vi "Save CRT data to file.vi"(5 "GPS data granularity (minutes)":refnum<vi>, 6 "Hitrate save info":T2, 7 "ROB data granularity (minutes)":refnum<vi>, 8 "error in":errorcluster, 9 "Run ID":refnum<vi>, 10 "ROB Info cluster":refnum<vi>, 11 "HDF5 data file":refnum<vi>) -> (0 "error out":errorcluster)   [LabVIEW 2016]
uses:
  Typedefs/Hit chart cluster refnum.ctl
  Typedefs/CoincidencesToSave.ctl
  Typedefs/CoincidenceWithGPSformat.ctl
  Global Variables/take CRT data.vi
  <vilib>/addons/h5labview2/group/H5G.lvlib
  <vilib>/addons/h5labview2/dataset/H5D.lvlib
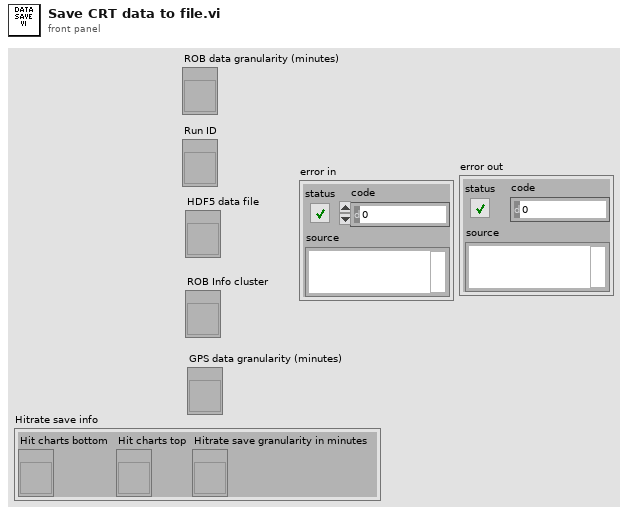
[diagram p1: front panel]
types:
  T1 = typedef "Hit chart cluster refnum.ctl" = refnum<vi>
  T2 = cluster{"Hit charts bottom":T1, "Hit charts top":T1, "Hitrate save granularity in minutes":refnum<vi>}
  T3 = typedef "CoincidenceWithGPSformat.ctl" = cluster{"Low-res hit time":u32, "Hi-res hit time":u32, "Secondary ID":i8, "DeltaT":i32, "Primary ID":i8}
  T4 = typedef "CoincidencesToSave.ctl" = T3[]
  T5 = cluster{"Timestamp":u32, "Fix quality":i8, "Satelites":i8}
  T6 = enum16{"insertPPS", "insertUTC", "read", "initiate"}
  T7 = typedef "hid_t.ctl" = i32
  T8 = cluster{"Pixel":i8, "Hi res hit time":u32, "Low res hit time":u32, "DeltaT":i16}[]
  T9 = typedef "HitChart.ctl" = cluster{"Waveform Chart":cluster{"Coincidences":dbl, "Non-coincidences":dbl, "Ratio":dbl, "Total hits":dbl}[], "Last update timestamp":timestamp, "Resolution(s)":dbl, "nondisplayed coincs":i32, "nondisplayed noncoincs":i32, "Last upd":i64, "ID":i8}
  T10 = cluster{"Waveform Chart":T9, "Waveform Chart 2":T9, "Waveform Chart 3":T9, "Waveform Chart 4":T9, "Waveform Chart 5":T9, "Waveform Chart 6":T9, "Waveform Chart 7":T9, "Waveform Chart 8":T9}
  T11 = cluster{"timestamp":u32, "ch0":dbl, "ch1":dbl, "ch2":dbl, "ch3":dbl, "ch4":dbl, "ch5":dbl, "ch6":dbl, "ch7":dbl, "ch8":dbl, "ch9":dbl, "ch10":dbl, "ch11":dbl, "ch12":dbl, "ch13":dbl, "ch14":dbl, "ch15":dbl}[]
  T12 = cluster{"Timestamp":u32, "Fix quality":i8, "Satelites":i8}[]
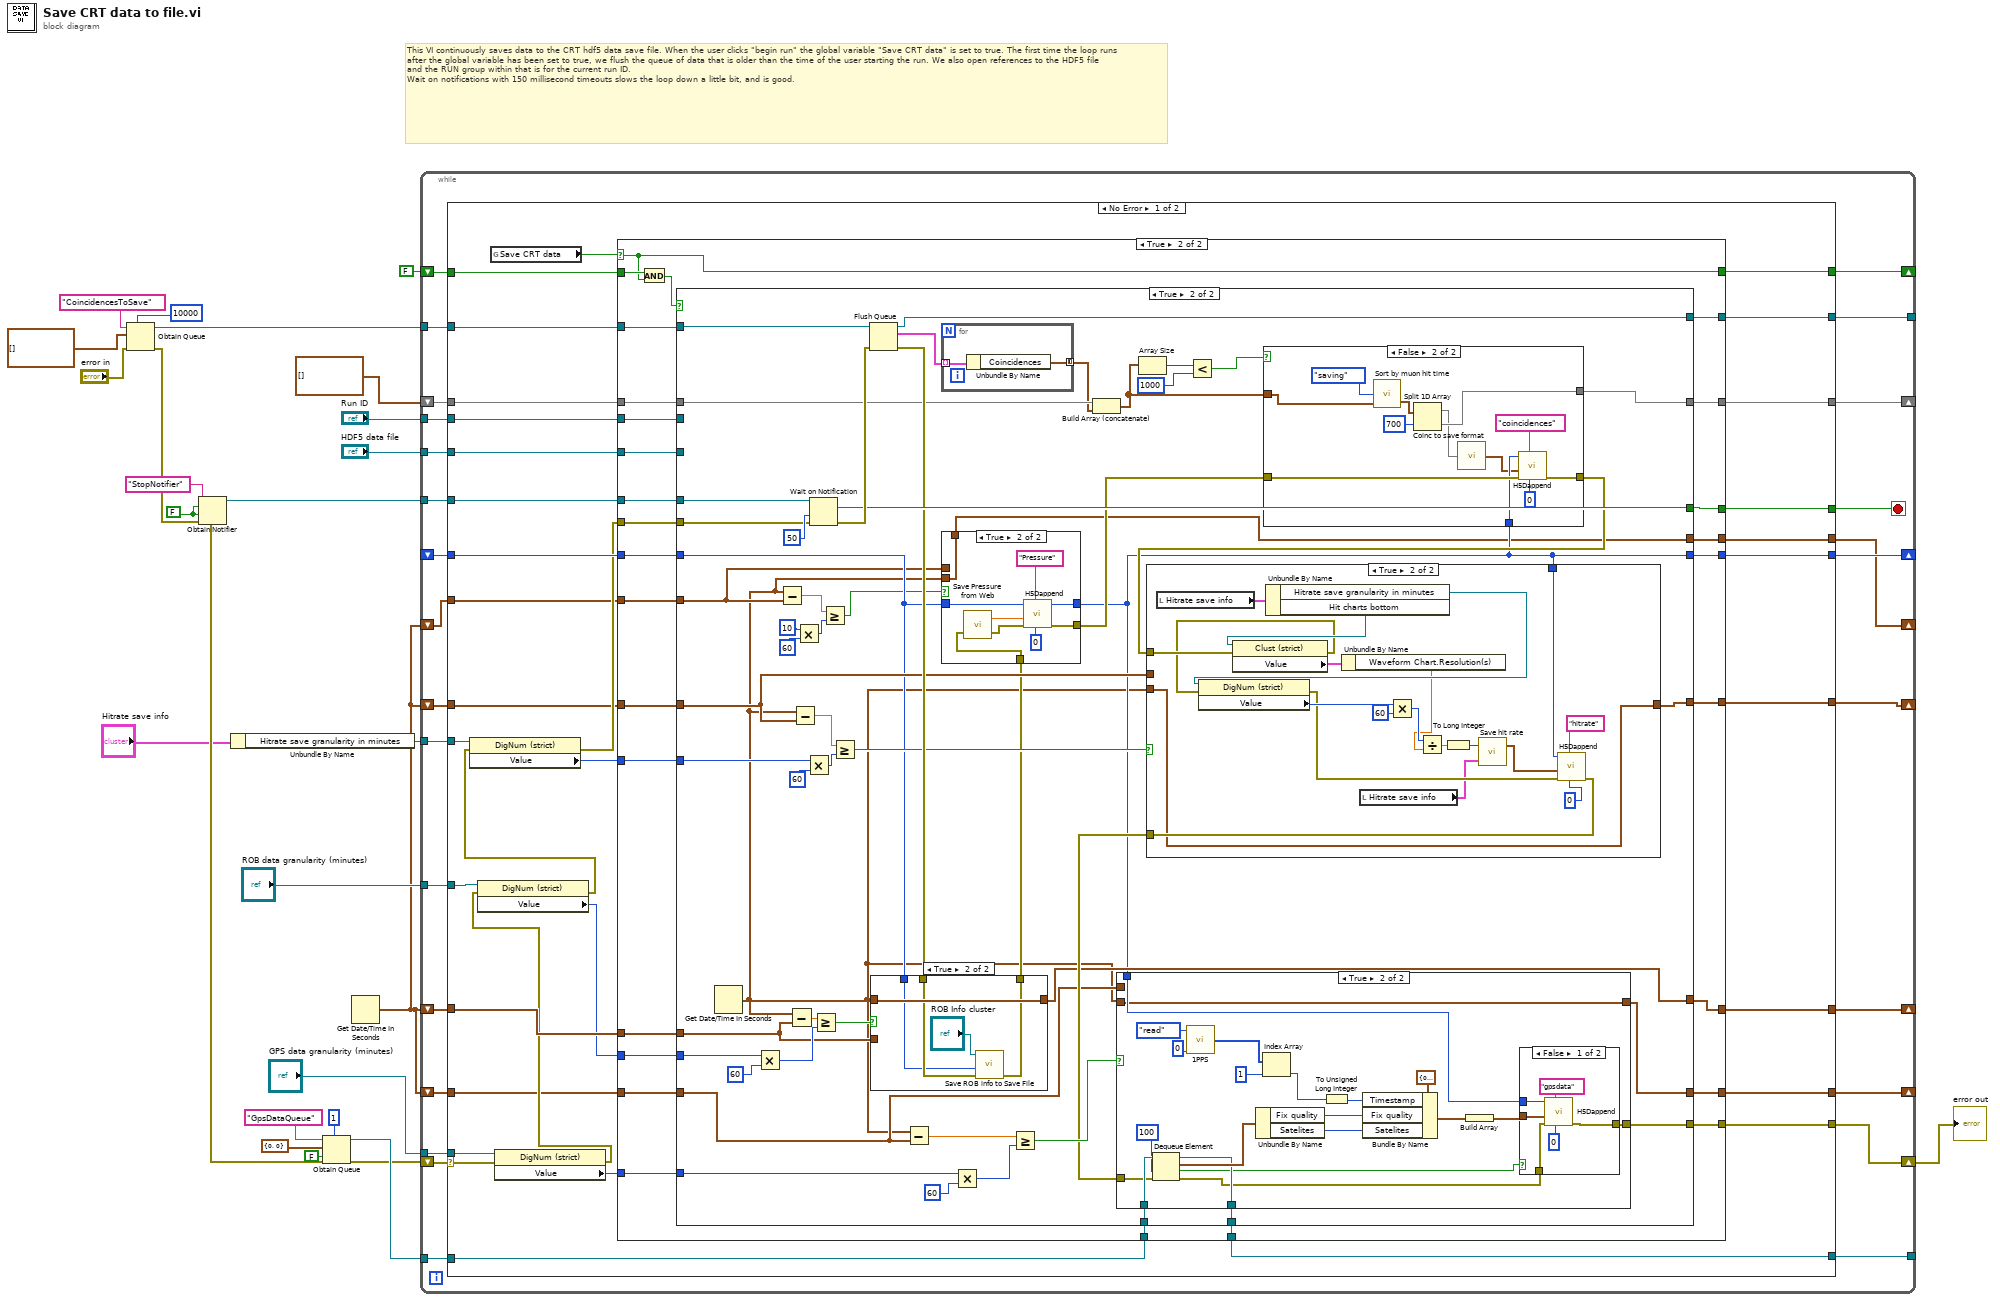
[diagram p0: block diagram]
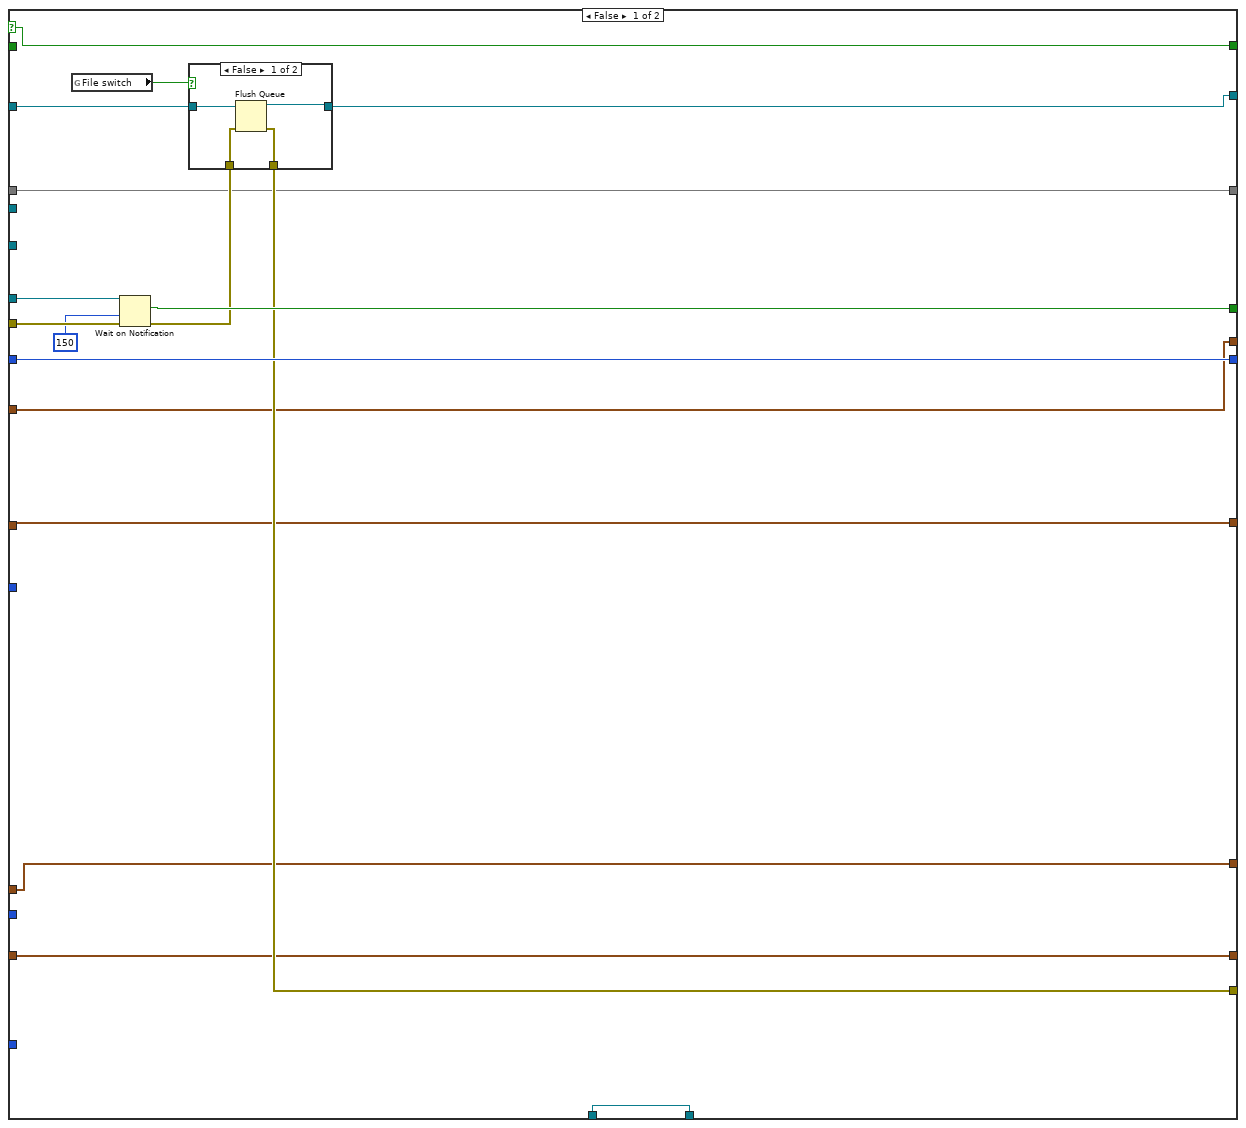
[diagram p2: hidden frame]
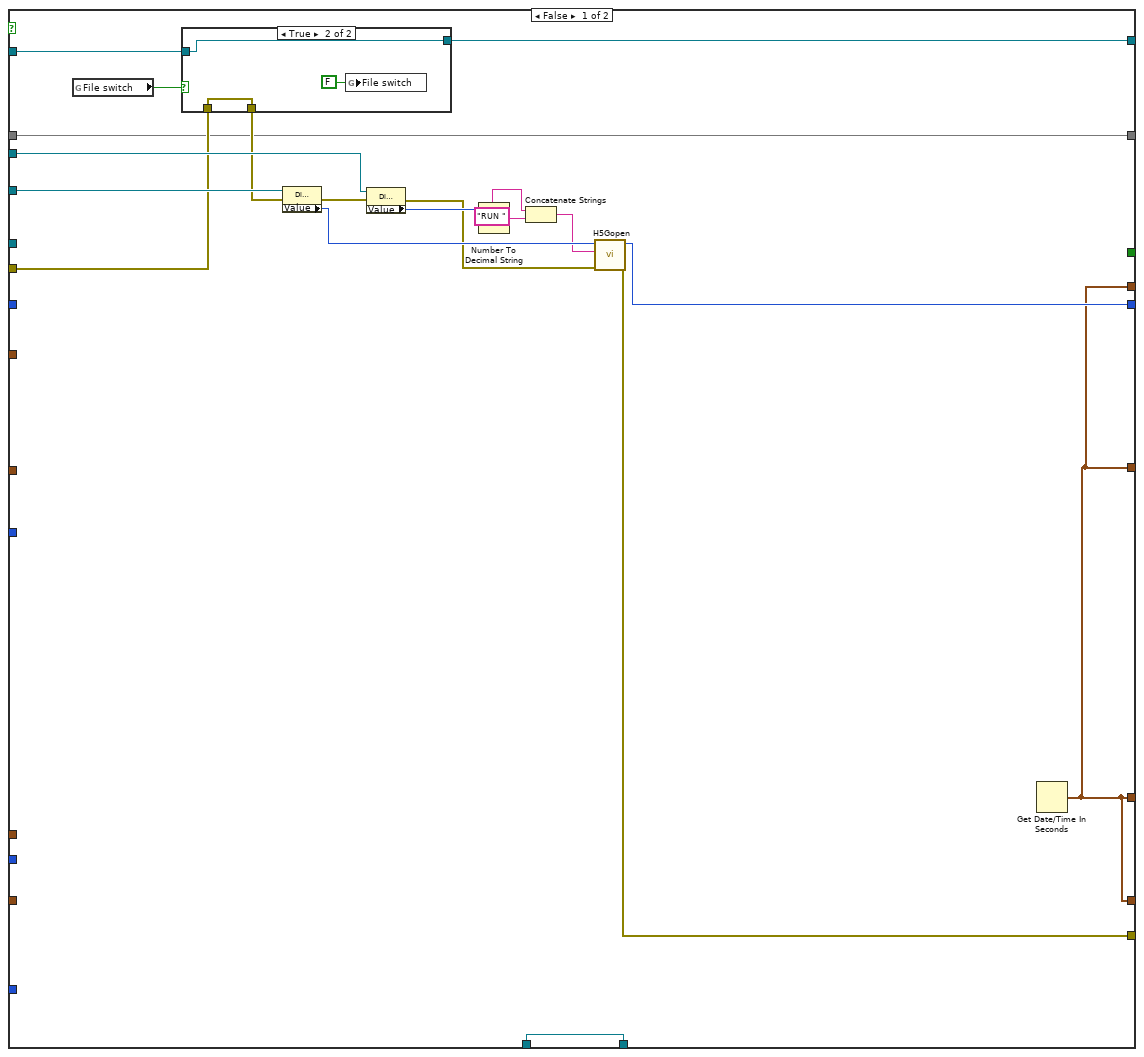
[diagram p4: hidden frame]
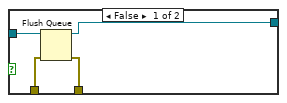
[diagram p5: hidden frame]
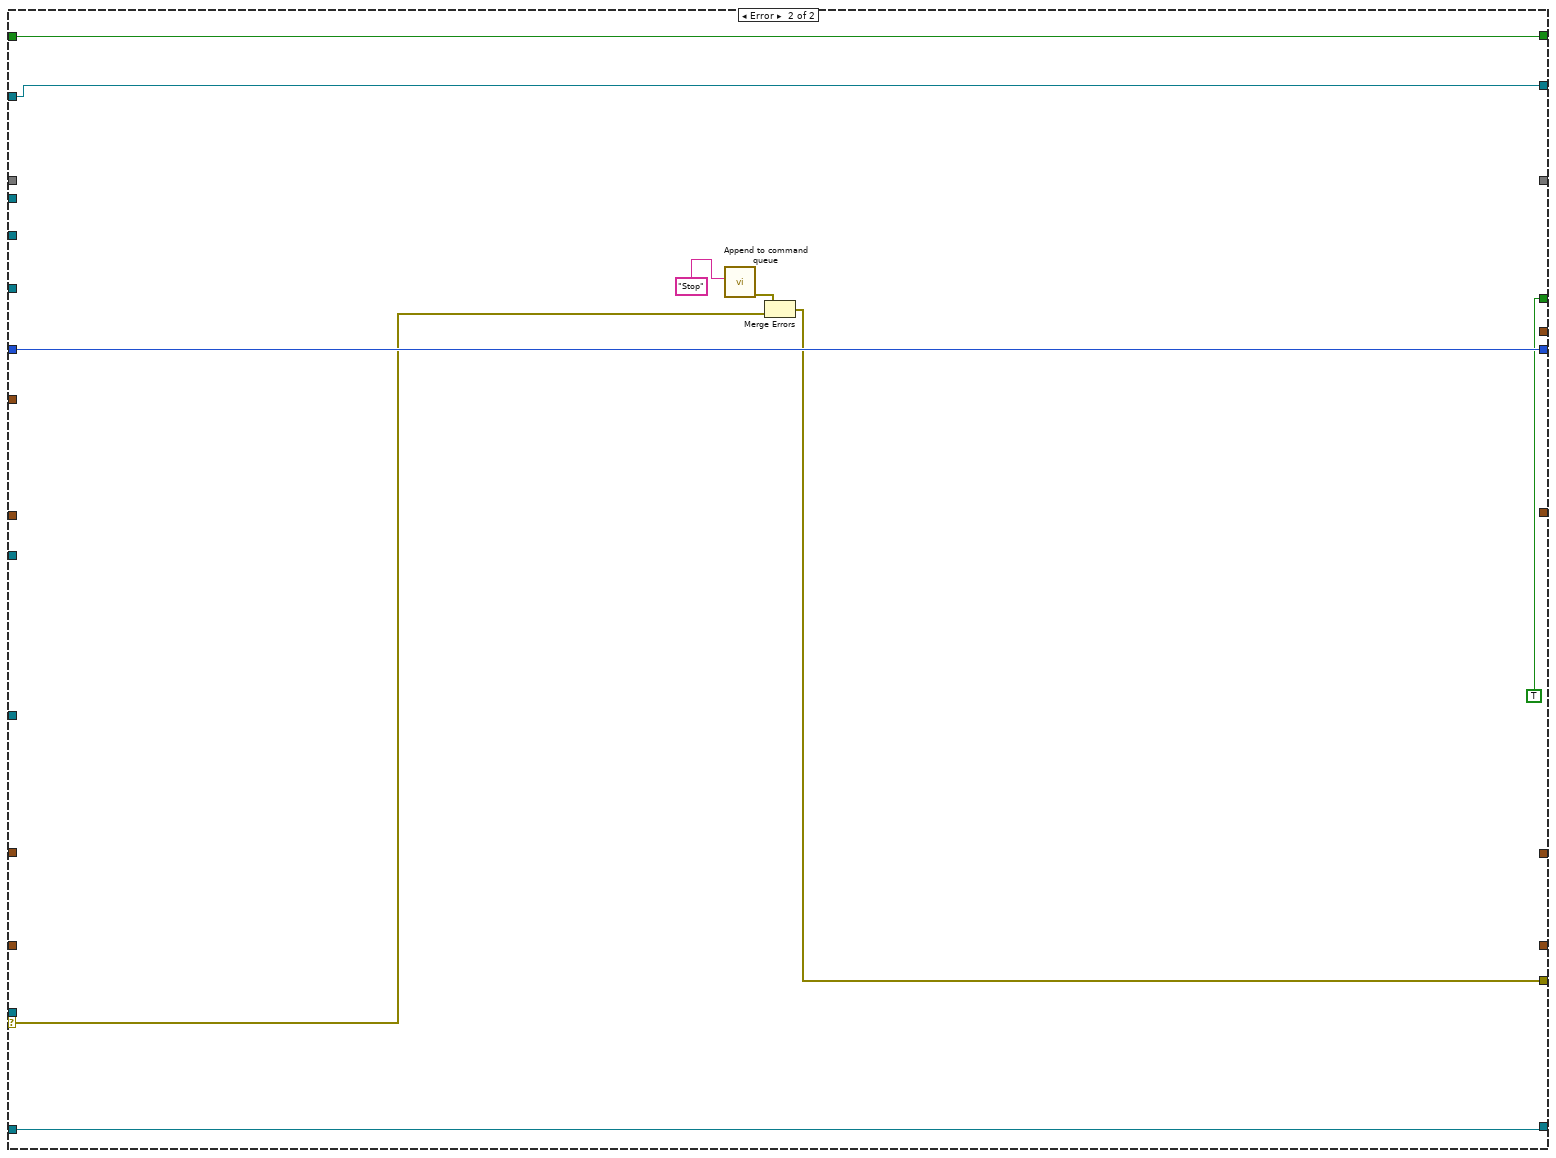
[diagram p12: hidden frame]
diagram:
  w19 = FALSE
  # "This VI continuously saves data to the CRT hdf5 data save file. When the user clicks \"begin run\" the global variable \"Save CRT data\" is set to true. The first time the loop runs after the global variable has been set to true, we flush the queue of data that is older than the time of the user starting the run. We also open references to the HDF5 file and the RUN group within that is for the current run ID.\nWait on notifications with 150 millisecond timeouts slows the loop down a little bit, and is good."
  n1 = Obtain Queue(max queue size (-1, unlimited)=10000, name (unnamed)="CoincidencesToSave", element data type=T4 [] ("Coincidences"), error in (no error)="error in") -> (queue out=w24:refnum<queue>, error out=w9:errorcluster)  [unwired: 1 in, 1 out]
  n2 = Obtain Notifier(name (unnamed)="StopNotifier", notification data type=w19, create if not found? (T)=w19, error in (no error)=w9) -> (notifier out=w18:refnum<notifier>, error out=w4:errorcluster)  [unwired: 1 out]
  n3 = Unbundle By Name("Hitrate save info") -> ("Hitrate save granularity in minutes"=w2:refnum<vi>)
  n4 = Obtain Queue(max queue size (-1, unlimited)=1, name (unnamed)="GpsDataQueue", element data type=cluster{"Fix quality":i8, "Satelites":i8} {"Fix quality"=0, "Satelites"=0}, create if not found? (T)=FALSE, error in (no error)=w4) -> (queue out=w8:refnum<queue>, error out=w6:errorcluster)  [unwired: 1 out]
  n5 = Get Date/Time In Seconds() -> (seconds since 1Jan1904=w1:timestamp)
  n6 = while {
    shift-right: [w53] -> _
    shift-left: FALSE -> [w52]
    tunnel: w24 -> [w51]
    shift-right: [w48] -> w17
    shift-left: w6 -> [w34]
    tunnel: "HDF5 data file" -> [w50]
    tunnel: "Run ID" -> [w49]
    shift-right: [w47] -> _
    shift-left: _ -> [w46]
    tunnel: w18 -> [w45]
    shift-right: [w41] -> _
    shift-left: w1 -> [w43]
    tunnel: "ROB data granularity (minutes)" -> [w42]
    shift-right: [w40] -> _
    shift-left: T3[] [] ("Coincidences") -> [w39]
    tunnel: "GPS data granularity (minutes)" -> [w38]
    tunnel: w8 -> [w37]
    tunnel: [w36] -> _
    tunnel: [w35] -> _
    tunnel: w2 -> [w33]
    shift-right: [w30] -> _
    shift-left: w1 -> [w32]
    shift-right: [w29] -> _
    shift-left: w1 -> [w31]
    shift-right: [w27] -> _
    shift-left: w1 -> [w28]
    stop <- w44 stop-if-true
    n7 = case shown="No Error" w34 {
      selector: w34 -> [w65 w311]
      tunnel: [w86 w314] -> w53
      tunnel: w52 -> [w85 w314]
      tunnel: w51 -> [w84 w307]
      tunnel: w50 -> [w83 _]
      tunnel: w49 -> [w82 _]
      tunnel: [w81 w310] -> w48
      tunnel: [w80 w315] -> w47
      tunnel: w46 -> [w79 w315]
      tunnel: w45 -> [w78 _]
      tunnel: [w77 TRUE] -> w44
      tunnel: w43 -> [w76 _]
      tunnel: w42 -> [w75 _]
      tunnel: [w73 _] -> w41
      tunnel: [w72 _] -> w40
      tunnel: w39 -> [w71 _]
      tunnel: w38 -> [w70 _]
      tunnel: w37 -> [w68 w308]
      tunnel: [w67 w307] -> w36
      tunnel: [w66 w308] -> w35
      tunnel: w33 -> [w63 _]
      tunnel: w32 -> [w59 _]
      tunnel: w31 -> [w58 _]
      tunnel: [w57 _] -> w30
      tunnel: [w56 _] -> w29
      tunnel: w28 -> [w55 _]
      tunnel: [w54 _] -> w27
      frame No Error {
        n8 = global read "take CRT data.vi" "Save CRT data"() -> (w87:bool)
        n9 = property class="DigNum (strict)"(reference=w70, error in=w65) -> (error out=w64:errorcluster, "Value"=w69:i32)  [unwired: 1 out]
        n10 = property class="DigNum (strict)"(reference=w75, error in=w64) -> (error out=w62:errorcluster, "Value"=w74:i32)  [unwired: 1 out]
        n11 = property class="DigNum (strict)"(reference=w63, error in=w62) -> (error out=w60:errorcluster, "Value"=w61:i32)  [unwired: 1 out]
        n12 = case shown="True" w87 {
          selector: w87 -> [w96 w137]
          tunnel: [w96 w137] -> w86
          tunnel: w85 -> [_ w138]
          tunnel: w84 -> [w99 w135]
          tunnel: w60 -> [w103 w134]
          tunnel: w83 -> [_ w133]
          tunnel: w82 -> [_ w132]
          tunnel: [w97 w131] -> w81
          tunnel: [w104 w130] -> w80
          tunnel: w79 -> [w104 w129]
          tunnel: w78 -> [w102 w128]
          tunnel: [w100 w127] -> w77
          tunnel: w76 -> [w95 w126]
          tunnel: w74 -> [_ w125]
          tunnel: [w95 w124] -> w73
          tunnel: [w94 w123] -> w72
          tunnel: w71 -> [w94 w122]
          tunnel: w69 -> [_ w121]
          tunnel: w68 -> [w92 w120]
          tunnel: [w91 w119] -> w67
          tunnel: [w92 w118] -> w66
          tunnel: w61 -> [_ w117]
          tunnel: w59 -> [w90 w116]
          tunnel: w58 -> [w89 w115]
          tunnel: [w90 w114] -> w57
          tunnel: [w89 w113] -> w56
          tunnel: w55 -> [w88 w112]
          tunnel: [w88 w111] -> w54
          frame False {
            n13 = global read "take CRT data.vi" "File switch"() -> (w93:bool)
            n14 = Wait on Notification(notifier=w102, timeout in ms (-1)=150, error in (no error)=w103) -> (notification=w100:bool, error out=w98:errorcluster)  [unwired: 1 in, 2 out]
            n15 = case shown="False" w93 {
              tunnel: w99 -> [w108 w109]
              tunnel: w98 -> [w107 w110]
              tunnel: [w106 w110] -> w97
              tunnel: [w105 w109] -> w91
              frame False {
                n16 = Flush Queue(queue=w108, error in (no error)=w107) -> (queue out=w105:refnum<queue>, error out=w106:errorcluster)  [unwired: 1 out]
              }
              frame True {
              }
            }
          }
          frame True {
            n17 = And(x=w138, y=w137) -> (x .and. y?=w136:bool)
            n18 = case shown="True" w136 {
              tunnel: w135 -> [w157 w218]
              tunnel: w134 -> [w146 w215]
              tunnel: w133 -> [w156 _]
              tunnel: w132 -> [w154 _]
              tunnel: [w144 w191] -> w131
              tunnel: [w147 w173] -> w130
              tunnel: w129 -> [_ w174]
              tunnel: w128 -> [_ w213]
              tunnel: [_ w212] -> w127
              tunnel: w126 -> [_ w196]
              tunnel: w125 -> [_ w211]
              tunnel: [w139 w181] -> w124
              tunnel: [w143 w204] -> w123
              tunnel: w122 -> [w143 w206]
              tunnel: w121 -> [_ w195]
              tunnel: w120 -> [w141 w194]
              tunnel: [w140 w193] -> w119
              tunnel: [w141 w192] -> w118
              tunnel: w117 -> [_ w189]
              tunnel: w116 -> [_ w179]
              tunnel: w115 -> [_ w177]
              tunnel: [w139 w180] -> w114
              tunnel: [w139 w178] -> w113
              tunnel: w112 -> [_ w167]
              tunnel: [w139 w166] -> w111
              frame False {
                n19 = global read "take CRT data.vi" "File switch"() -> (w142:bool)
                n20 = case shown="True" w142 {
                  tunnel: w157 -> [w161 w162]
                  tunnel: w146 -> [w160 w164]
                  tunnel: [w159 w164] -> w145
                  tunnel: [w158 w162] -> w140
                  frame False {
                    n21 = Flush Queue(queue=w161, error in (no error)=w160) -> (queue out=w158:refnum<queue>, error out=w159:errorcluster)  [unwired: 1 out]
                  }
                  frame True {
                    n22 = global write "take CRT data.vi" "File switch"(FALSE ("File switch")) -> ()
                  }
                }
                n23 = property class="DigNum (strict)"(reference=w156, error in=w145) -> (error out=w155:errorcluster, "Value"=w153:T7)  [unwired: 1 out]
                n24 = property class="DigNum (strict)"(reference=w154, error in=w155) -> (error out=w148:errorcluster, "Value"=w152:i32)  [unwired: 1 out]
                n25 = Number To Decimal String(number=w152) -> (decimal integer string=w150:string)  [unwired: 1 in]
                n26 = Concatenate Strings("RUN ", w150) -> (w149:string)
                n27 = call <vilib>:"H5Gopen.vi"("error in (no error)"=w148, "name"=w149, "ref in"=w153) -> ("error out"=w144:errorcluster, "group out"=w147:T7)  [unwired: 7 in]
                n28 = Get Date/Time In Seconds() -> (seconds since 1Jan1904=w139:timestamp)
              }
              frame True {
                n29 = Get Date/Time In Seconds() -> (seconds since 1Jan1904=w165:timestamp)
                n30 = Multiply(x=w211, y=60) -> (x*y=w209:i32)
                n31 = Subtract(x=w165, y=w167) -> (x-y=w172:dbl)
                n32 = Subtract(x=w165, y=w196) -> (x-y=w184:dbl)
                n33 = Subtract(x=w165, y=w177) -> (x-y=w182:dbl)
                n34 = Multiply(x=10, y=60) -> (x*y=w171:i32)
                n35 = Multiply(x=w189, y=60) -> (x*y=w188:i32)
                n36 = Wait on Notification(notifier=w213, timeout in ms (-1)=50, error in (no error)=w215) -> (notification=w212:bool, error out=w214:errorcluster)  [unwired: 1 in, 2 out]
                n37 = Greater Or Equal?(x=w184, y=w209) -> (x >= y?=w207:bool)
                n38 = Greater Or Equal?(x=w172, y=w171) -> (x >= y?=w168:bool)
                n39 = Greater Or Equal?(x=w182, y=w188) -> (x >= y?=w187:bool)
                n40 = Flush Queue(queue=w218, error in (no error)=w214) -> (queue out=w193:refnum<queue>, remaining elements=w217:cluster{"Coincidences":T4}[], error out=w208:errorcluster)
                n41 = case shown="True" w207 {
                  tunnel: w208 -> [w285 w287]
                  tunnel: w174 -> [_ w286]
                  tunnel: [w285 w288] -> w176
                  tunnel: w165 -> [_ w289]
                  tunnel: w196 -> [w284 _]
                  tunnel: [w284 w289] -> w181
                  frame False {
                  }
                  frame True {
                    n42 = call "Save ROB info to Save File.vi"("error in (no error)"=w287, "Fileref"=w286, "ROB info clusters"="ROB Info cluster") -> ("error out"=w288:errorcluster)  [unwired: 8 in]
                  }
                }
                n43 = Subtract(x=w165, y=w179) -> (x-y=w183:dbl)
                n44 = for {
                  tunnel: w217 -> [w306] mode=indexing
                  tunnel: [w305] -> w205 mode=concatenating
                  n45 = Unbundle By Name(w306) -> ("Coincidences"=w305:T4)
                }
                n46 = case shown="True" w168 {
                  tunnel: w176 -> [w220 w230]
                  tunnel: [w220 w226] -> w175
                  tunnel: w174 -> [w221 w224]
                  tunnel: [w221 w223] -> w173
                  tunnel: w167 -> [w219 _]
                  tunnel: [w219 w222] -> w166
                  tunnel: w165 -> [_ w222]
                  frame False {
                  }
                  frame True {
                    n47 = call "Save Pressure from Web.vi"("error in"=w230) -> ("error out"=w227:errorcluster, "Pressure"=w229:dbl)  [unwired: 1 in]
                    n48 = call <vilib>:"H5Dappend.vi"("axis (first)"=0, "dataset name"="Pressure", "error in (no error)"=w227, "data"=w229, "ref in"=w224) -> ("error out"=w226:errorcluster, "ref out"=w223:T7)  [unwired: 3 in, 2 out]
                  }
                }
                n49 = Multiply(x=w195, y=60) -> (x*y=w199:i32)
                n50 = Greater Or Equal?(x=w183, y=w199) -> (x >= y?=w197:bool)
                n51 = Build Array (concatenate)(w206, w205) -> (w203:T4)
                n52 = Array Size(array=w203) -> (size(s)=w202:i32)
                n53 = Less?(x=w202, y=1000) -> (x < y?=w200:bool)
                n54 = case shown="False" w200 {
                  tunnel: w175 -> [w292 w304]
                  tunnel: [w292 w303] -> w185
                  tunnel: w173 -> [_ w302]
                  tunnel: [w291 w297] -> w204
                  tunnel: w203 -> [w291 w294]
                  frame True {
                  }
                  frame False {
                    n55 = call "Sort by muon hit time.vi"("Top Coincs saving"=w294, "Type"=enum16{"internal", "saving"}."saving") -> ("Coincidences saving"=w298:T4)  [unwired: 1 in, 1 out]
                    n56 = Split 1D Array(array=w298, index=700) -> (first subarray=w296:T4, second subarray=w297:T4)
                    n57 = call "Coinc to save format.vi"("Coincidences"=w296) -> ("Array"=w295:T8)
                    n58 = call <vilib>:"H5Dappend.vi"("axis (first)"=0, "dataset name"="coincidences", "error in (no error)"=w304, "data"=w295, "ref in"=w302) -> ("error out"=w303:errorcluster)  [unwired: 3 in, 3 out]
                  }
                }
                n59 = case shown="True" w187 {
                  tunnel: [w232 w242] -> w186
                  tunnel: w173 -> [_ w241]
                  tunnel: w185 -> [w232 w237]
                  tunnel: [w231 w234] -> w178
                  tunnel: w177 -> [w231 _]
                  tunnel: w165 -> [_ w234]
                  frame False {
                  }
                  frame True {
                    n60 = local read "Hitrate save info"() -> (w247:T2)
                    n61 = Unbundle By Name(w247) -> ("Hitrate save granularity in minutes"=w252:refnum<vi>, "Hit charts bottom"=w240:T1)
                    n62 = property class="Clust (strict)"(reference=w240, error in=w237) -> (error out=w236:errorcluster, "Value"=w239:T10)  [unwired: 1 out]
                    n63 = property class="DigNum (strict)"(reference=w252, error in=w236) -> (error out=w235:errorcluster, "Value"=w251:i32)  [unwired: 1 out]
                    n64 = Unbundle By Name(w239) -> ("Waveform Chart.Resolution(s)"=w238:dbl)
                    n65 = local read "Hitrate save info"() -> (w233:T2)
                    n66 = Multiply(x=w251, y=60) -> (x*y=w249:i32)
                    n67 = Divide(x=w249, y=w238) -> (x/y=w248:dbl)
                    n68 = To Long Integer(number=w248) -> (32bit integer=w246:i32)
                    n69 = call "Save hit rate.vi"("Data cluster"=w233, "Elements to average"=w246) -> ("data"=w243:T11)  [unwired: 1 in]
                    n70 = call <vilib>:"H5Dappend.vi"("axis (first)"=0, "dataset name"="hitrate", "error in (no error)"=w235, "data"=w243, "ref in"=w241) -> ("error out"=w242:errorcluster)  [unwired: 3 in, 3 out]
                  }
                }
                n71 = case shown="True" w197 {
                  tunnel: [w253 w256] -> w180
                  tunnel: w165 -> [_ w256]
                  tunnel: w173 -> [_ w263]
                  tunnel: w186 -> [w255 w271]
                  tunnel: [w255 w268] -> w191
                  tunnel: w194 -> [w254 w272]
                  tunnel: [w254 w269] -> w192
                  tunnel: w179 -> [w253 _]
                  frame False {
                  }
                  frame True {
                    n72 = Dequeue Element(queue=w272, timeout in ms (-1)=100, error in (no error)=w271) -> (queue out=w269:refnum<queue>, element=w270:cluster{"Fix quality":i8, "Satelites":i8}, timed out?=w261:bool, error out=w264:errorcluster)
                    n73 = call "1PPS.vi"("Read Index\nNumber"=0 ("Read Index\nNumber"), "Action"=T6."read") -> ("Array"=w276:u32[])  [unwired: 2 in]
                    n74 = Unbundle By Name(w270) -> ("Fix quality"=w267:i8, "Satelites"=w266:i8)
                    n75 = Index Array(array=w276, index=1) -> (element=w258:u32)
                    n76 = To Unsigned Long Integer(number=w258) -> (unsigned 32bit integer=w257:u32)
                    n77 = Bundle By Name(cluster=T5 {"Timestamp"=0, "Fix quality"=0, "Satelites"=0} ("output cluster"), "Timestamp"=w257, "Fix quality"=w267, "Satelites"=w266) -> (w260:T5)
                    n78 = Build Array(w260) -> (w259:T12)
                    n79 = case shown="False" w261 {
                      tunnel: [w281 w283] -> w268
                      tunnel: w259 -> [w280 _]
                      tunnel: w264 -> [w279 w283]
                      tunnel: w263 -> [w278 _]
                      frame False {
                        n80 = call <vilib>:"H5Dappend.vi"("axis (first)"=0, "dataset name"="gpsdata", "error in (no error)"=w279, "data"=w280, "ref in"=w278) -> ("error out"=w281:errorcluster)  [unwired: 3 in, 3 out]
                      }
                      frame True {
                      }
                    }
                  }
                }
              }
            }
          }
        }
      }
      frame Error {
        n81 = call "Append to command queue.vi"("Single command"="Stop") -> ("error out"=w312:errorcluster)  [unwired: 10 in]
        n82 = Merge Errors(w312, w311) -> (w310:errorcluster)
      }
    }
  }
  "error out" <- w17
